vi "GLOBALHarvester.vi"() -> ()   [LabVIEW 2011]
panel:
  out "Harvester Output":dbl
  out "Conveyor Output":dbl
  out "Balls In Robot":dbl
  out "SP3 Process":bool
  out "SP12 Process":bool
  in  "Shoot":bool
  in  "SP 3":bool
  in  "SP 2":bool
  in  "SP 1":bool
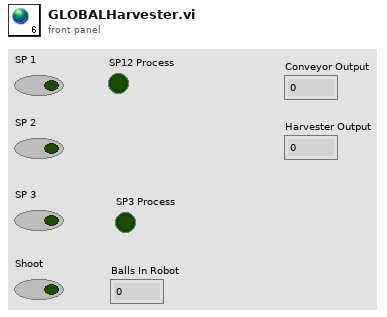
[diagram p1: front panel]
diagram:
